vi "BMark_PositionHelpLink.vi"(8 "error in (no error)":errorcluster, 10 "More information":refnum<vi>, 11 "Warning glyph":refnum<vi>) -> (0 "error out":errorcluster)   [LabVIEW 2018]
uses:
  globals/BMark_User Visible Strings.vi
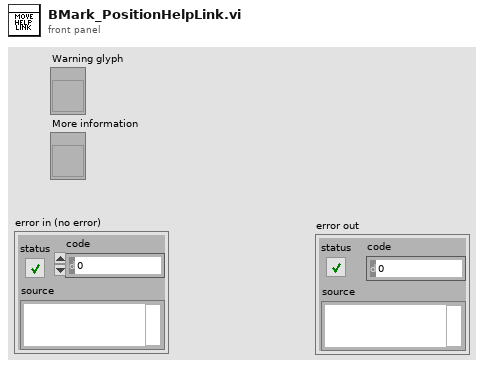
[diagram p1: front panel]
types:
  T1 = typedef "LVPointTypeDef.ctl" = cluster{"Horizontal":i16, "Vertical":i16}
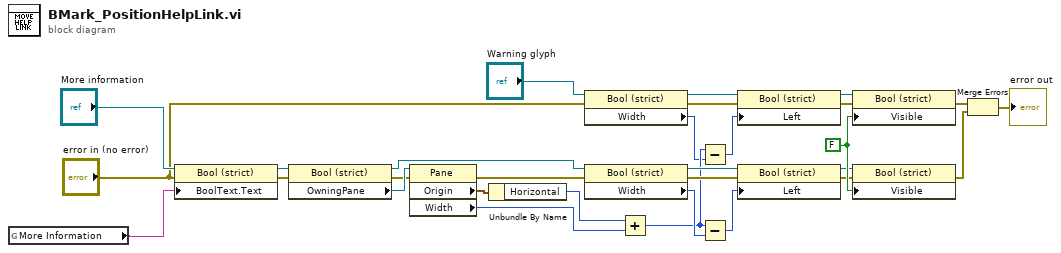
[diagram p0: block diagram]
diagram:
  w8 = FALSE ("Visible")
  n1 = global read "BMark_User Visible Strings.vi" "More Information"() -> (w1:string)
  n2 = property class="Bool (strict)"(reference="More information", error in="error in (no error)", "BoolText.Text"=w1) -> (reference out=w18:refnum<vi>, error out=w17:errorcluster)
  n3 = property class="Bool (strict)"(reference=w18, error in=w17) -> (reference out=w30:refnum<vi>, error out=w22:errorcluster, "OwningPane"=w29:refnum<vi>)
  n4 = property class="Pane"(reference=w29, error in=w22) -> (error out=w21:errorcluster, "Origin"=w28:T1, "Width"=w26:u32)  [unwired: 1 out]
  n5 = Unbundle By Name(w28) -> ("Horizontal"=w27:i16)
  n6 = property class="Bool (strict)"(reference="Warning glyph", error in="error in (no error)") -> (reference out=w13:refnum<vi>, error out=w12:errorcluster, "Width"=w15:u32)
  n7 = property class="Bool (strict)"(reference=w30, error in=w21) -> (reference out=w24:refnum<vi>, error out=w20:errorcluster, "Width"=w25:u32)
  n8 = Add(x=w27, y=w26) -> (x+y=w16:u32)
  n9 = Subtract(x=w16, y=w15) -> (x-y=w14:u32)
  n10 = Subtract(x=w16, y=w25) -> (x-y=w23:u32)
  n11 = property class="Bool (strict)"(reference=w13, error in=w12, "Left"=w14) -> (reference out=w7:refnum<vi>, error out=w5:errorcluster)
  n12 = property class="Bool (strict)"(reference=w24, error in=w20, "Left"=w23) -> (reference out=w6:refnum<vi>, error out=w4:errorcluster)
  n13 = property class="Bool (strict)"(reference=w7, error in=w5, "Visible"=w8) -> (error out=w3:errorcluster)  [unwired: 1 out]
  n14 = property class="Bool (strict)"(reference=w6, error in=w4, "Visible"=w8) -> (error out=w2:errorcluster)  [unwired: 1 out]
  n15 = Merge Errors(w3, w2) -> (→"error out":errorcluster)
